vi "Pod Drawing Utility.vi"() -> (3 "Cluster":cluster{dbl[], dbl[]})   [LabVIEW 2025]
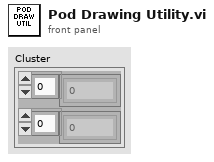
[diagram p1: front panel]
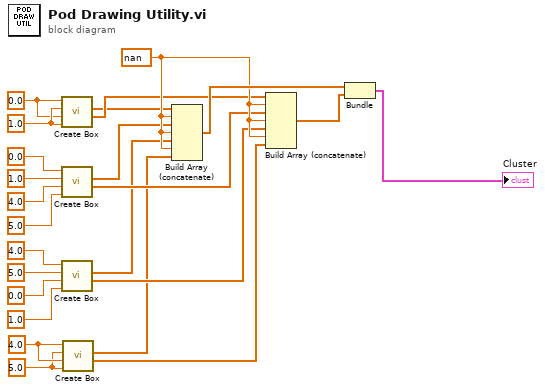
[diagram p0: block diagram]
diagram:
  w21 = nan ("Left")
  w11 = 5.0 ("Right")
  w12 = 4.0 ("Left")
  w2 = 1.0 ("Right")
  w1 = 0.0 ("Left")
  n1 = call "Create Box.vi"("Top"=w2, "Bottom"=w1, "Right"=w2, "Left"=w1) -> ("Y"=w17:dbl[], "X"=w13:dbl[])  [unwired: 5 in, 1 out]
  n2 = call "Create Box.vi"("Top"=5.0, "Bottom"=4.0, "Right"=1.0, "Left"=0.0) -> ("Y"=w18:dbl[], "X"=w14:dbl[])  [unwired: 5 in, 1 out]
  n3 = call "Create Box.vi"("Top"=1.0, "Bottom"=0.0, "Right"=5.0, "Left"=4.0) -> ("Y"=w19:dbl[], "X"=w15:dbl[])  [unwired: 5 in, 1 out]
  n4 = call "Create Box.vi"("Top"=w11, "Bottom"=w12, "Right"=w11, "Left"=w12) -> ("Y"=w20:dbl[], "X"=w16:dbl[])  [unwired: 5 in, 1 out]
  n5 = Build Array (concatenate)(w13, w21, w14, w21, w15, w21, w16) -> (w23:dbl[])
  n6 = Build Array (concatenate)(w17, w21, w18, w21, w19, w21, w20) -> (w22:dbl[])
  n7 = Bundle(w23, w22) -> (→"Cluster":cluster{dbl[], dbl[]})  [unwired: 1 in]
